vi "captureSpectImage.vi"(0 "ContextThisComponent in":refnum<class "ContextThisComponent.lvclass">, 1 "spectId":u16, 2 "intTime":sgl, 3 "intDelay":dbl, 4 "numAverages":u16, 5 "error in (no error)":errorcluster, 6 "CommandID":i32, 7 "numScans":i32, 9 "type":string, 11 "lamp":string) -> (14 "ContextThisComponent out":refnum<class "ContextThisComponent.lvclass">, 19 "error out":errorcluster)   [LabVIEW 2016, in "ContextThisComponent.lvclass"]
uses:
  ContextThisComponent.lvclass
  State/State.lvclass
  IStateFactory/IStateFactory.lvclass
  IModel/IModel.lvclass
  ts_sallv_sedspectrometer/DataTypes/command_captureSpectImage.ctl
  ts_sallv_sedspectrometer/SALLV_sedSpectrometer.lvlib
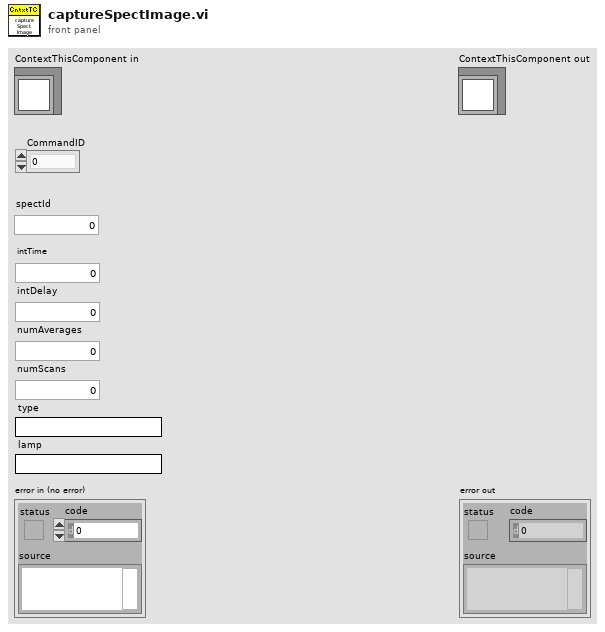
[diagram p1: front panel]
types:
  T1 = typedef "SALLV_sedSpectrometer.lvlib/command_captureSpectImage.ctl" = cluster{"spectId":u16, "intTime":sgl, "intDelay":dbl, "numAverages":u16, "numScans":i32, "type":string, "lamp":string}
  T2 = typedef "SALLV_sedSpectrometer.lvlib/logevent_DetailedState.ctl" = cluster{"detailedState":enum16{"", "DisabledState", "EnabledState", "FaultState", "OfflineState", "StandbyState", "CapturingSpectImage", "NotImaging"}, "priority":i32}
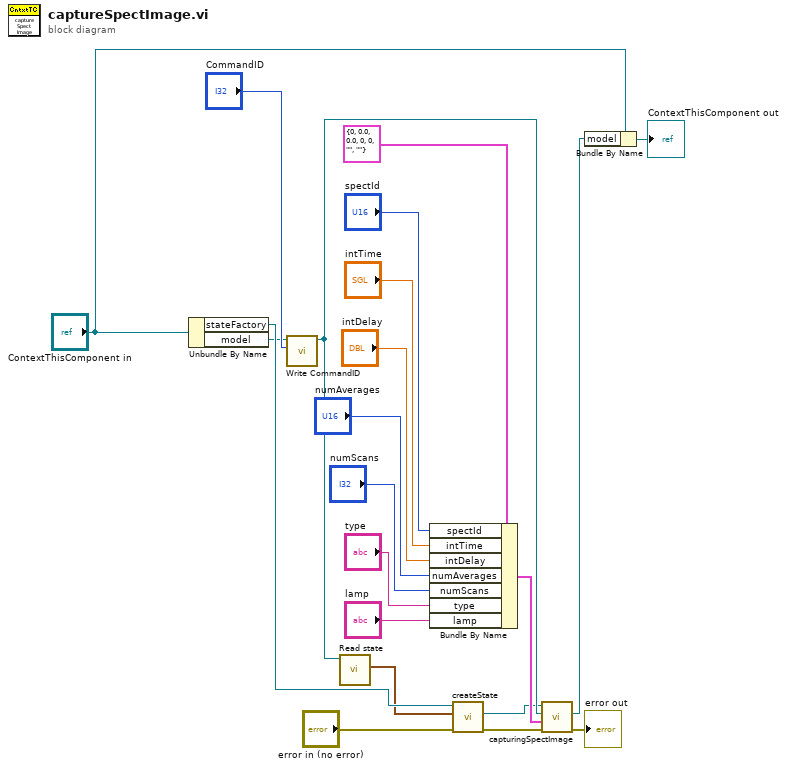
[diagram p0: block diagram]
diagram:
  n1 = Unbundle By Name("ContextThisComponent in") -> ("stateFactory"=w21:refnum<class "IStateFactory.lvclass">, "model"=w19:refnum<class "IModel.lvclass">)
  n2 = call-dynamic "Write CommandID.vi"("CommandID"="CommandID", "IModel in"=w19) -> ("IModel out"=w6:refnum<class "IModel.lvclass">)  [unwired: 8 in, 1 out]
  n3 = call-dynamic "Read state.vi"("IModel in"=w6) -> ("DetailedState"=w18:T2)  [unwired: 9 in, 1 out]
  n4 = Bundle By Name(cluster=T1 {"spectId"=0, "intTime"=0.0, "intDelay"=0.0, "numAverages"=0, "numScans"=0, "type"="", "lamp"=""} ("command_captureSpectImage"), "spectId"="spectId", "intTime"="intTime", "intDelay"="intDelay", "numAverages"="numAverages", "numScans"="numScans", "type"="type", "lamp"="lamp") -> (w7:T1)
  n5 = call-dynamic "createState.vi"("error in (no error)"="error in (no error)", "DetailedState"=w18, "IStateFactory in"=w21) -> ("error out"=w16:errorcluster, "state"=w5:refnum<class "State.lvclass">)  [unwired: 6 in, 1 out]
  n6 = call-dynamic "capturingSpectImage.vi"("error in (no error)"=w16, "command_captureSpectImage"=w7, "model in"=w6, "State in"=w5) -> ("error out"=→"error out":errorcluster, "model out"=w4:refnum<class "IModel.lvclass">)  [unwired: 5 in, 1 out]
  n7 = Bundle By Name(cluster="ContextThisComponent in", "model"=w4) -> (→"ContextThisComponent out":refnum<class "ContextThisComponent.lvclass">)
